vi "tools_openExampleFolder.vi"   [LabVIEW 2023]
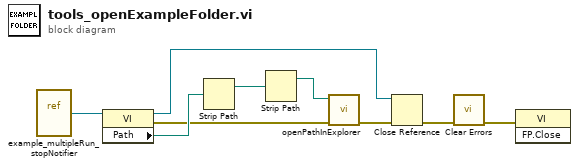
[diagram p0: block diagram]
diagram:
  n1 = vi-ref "example_multipleRun_stopNotifier.vi"() -> (w9:refnum<vi>)
  n2 = property class="VI"(reference=w9) -> (reference out=w4:refnum<vi>, error out=w5:errorcluster, "Path"=w8:path)  [unwired: 1 in]
  n3 = Strip Path(path=w8) -> (stripped path=w7:path)  [unwired: 1 out]
  n4 = Strip Path(path=w7) -> (stripped path=w6:path)  [unwired: 1 out]
  n5 = call "openPathInExplorer.vi"("error in (no error)"=w5, "pathToOpen"=w6) -> ("error out"=w3:errorcluster)  [unwired: 9 in]
  n6 = Close Reference(reference=w4, error in (no error)=w3) -> (error out=w2:errorcluster)
  n7 = call <vilib>:"Clear Errors.vi"("error in (no error)"=w2) -> ("error out"=w1:errorcluster)  [unwired: 5 in, 1 out]
  n8 = invoke class="VI" method="FP.Close"(error in=w1) -> ()  [unwired: 2 in, 3 out]
